vi "SECoP_dataCreateScaled.vi"(6 "value":i64, 7 "scale factor":dbl=1.0, 8 "error in (no error)":errorcluster, 9 "maximum value":i64=9223372036854775807, 10 "minimum value":i64=-9223372036854775807, 11 "DLL path (in)":T2) -> (0 "error out":errorcluster, 2 "SECoP_dataPtr (out)":T1 {"ptr64" format="%.0x"; "ptr32" format="%.0x"}, 3 "DLL path (out)":T2)   [LabVIEW 2023, in "SECoP.lvlib"]
doc: "Call <b>\"SECoP_dataCreateScaled.vi\"</b> to create a simple scaled (numeric) data type and set value. This data type is based on an integer with a scaling factor. Free resources after use with <b>\"SECoP_dataDestroy.vi\"</b>.\n\n<b>DLL path</b> input and output of cluster from \"SECoP-Initialize.vi\"\n<b>scale factor</b> scaling factor\n<b>minimum value</b> smallest allowed integer value without scaling\n<b>maximum value</b> greatest allowed integer value without scaling\n<b>value</b> new value\n<b>SECoP_dataPtr</b> created data"
uses:
  SECoP.lvlib
  SECoP-libraries.ctl
  SECoP-data.ctl
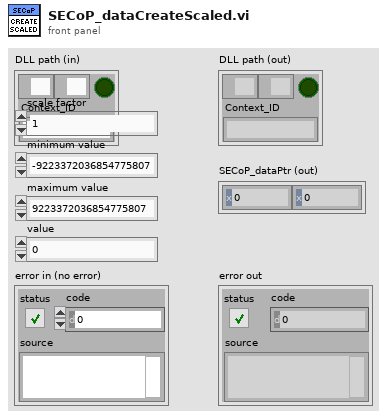
[diagram p1: front panel]
types:
  T1 = typedef "SECoP.lvlib/SECoP-data.ctl" = cluster{"ptr32":u32, "ptr64":u64}
  T2 = typedef "SECoP.lvlib/SECoP-libraries.ctl" = cluster{"serverDLL":path, "variantDLL":path, "cleanup_mode":bool, "Context_ID":string}
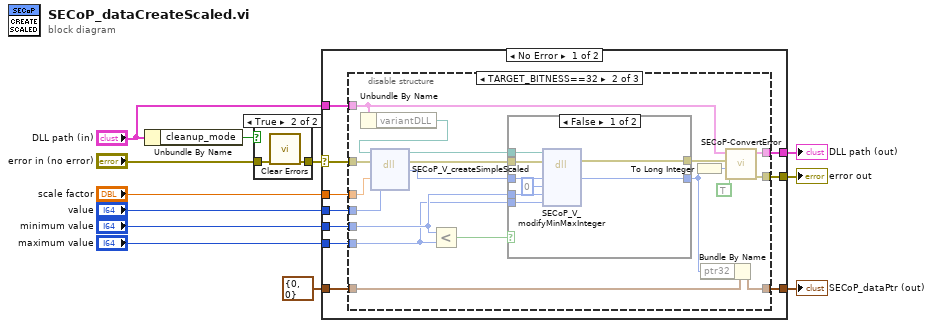
[diagram p0: block diagram]
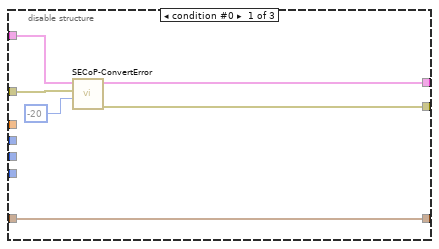
[diagram p3: hidden frame]
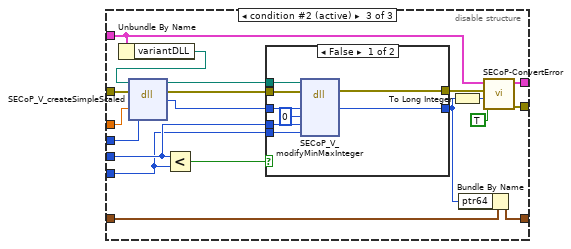
[diagram p5: hidden frame]
diagram:
  n1 = Unbundle By Name("DLL path (in)") -> ("cleanup_mode"=w10:bool)
  n2 = case shown="True" w10 {
    tunnel: "error in (no error)" -> [w13 w15]
    tunnel: [w13 w14] -> w8
    frame False {
    }
    frame True {
      n3 = call <vilib>:"Clear Errors.vi"("error in (no error)"=w15) -> ("error out"=w14:errorcluster)  [unwired: 5 in, 1 out]
    }
  }
  n4 = case shown="No Error" w8 {
    selector: w8 -> [w25 w91]
    tunnel: "DLL path (in)" -> [w24 w92]
    tunnel: [w22 w92] -> w12
    tunnel: [w23 w91] -> w11
    tunnel: [w20 w90] -> w7
    tunnel: T1 {"ptr32"=0, "ptr64"=0} ("SECoP_dataPtr (out)") -> [w21 w90]
    tunnel: "minimum value" -> [w19 _]
    tunnel: "maximum value" -> [w18 _]
    tunnel: "scale factor" -> [w17 _]
    tunnel: "value" -> [w16 _]
    frame No Error {
      n5 = disable-structure shown="TARGET_BITNESS==32" {
        disable-tunnel: w25 -> [w31 w50 w79]
        disable-tunnel: w24 -> [w30 w33 w62]
        disable-tunnel: [w28 w47 w76] -> w23
        disable-tunnel: [w29 w46 w75] -> w22
        disable-tunnel: w21 -> [w26 w48 w77]
        disable-tunnel: [w26 w49 w78] -> w20
        disable-tunnel: w19 -> [_ w38 w67]
        disable-tunnel: w18 -> [_ w37 w66]
        disable-tunnel: w17 -> [_ w35 w64]
        disable-tunnel: w16 -> [_ w34 w63]
        frame condition #0 {
          n6 = call "SECoP-ConvertError.vi"("return code"=-20, "error in (no error)"=w31, "DLL path (in)"=w30) -> ("error out"=w28:errorcluster, "DLL path (out)"=w29:T2)  [unwired: 7 in]
        }
        frame condition #1 {
          n7 = Unbundle By Name(w33) -> ("variantDLL"=w32:path)
          n8 = dll-call lib="Z:/Praktische_Aufgaben/SECoP-LabVIEW2015/32bit/SECoP32.dll" fn="SECoP_V_createSimpleScaled"(path in=w32, error in=w50, "dScale"=w35, "llValue"=w34) -> (path out=w43:path, error out=w42:errorcluster, "return type"=w40:u32)  [unwired: 3 in]
          n9 = Less?(x=w38, y=w37) -> (x < y?=w36:bool)
          n10 = case shown="False" w36 {
            tunnel: w43 -> [w58 _]
            tunnel: w42 -> [w57 w60]
            tunnel: [w56 w60] -> w41
            tunnel: w40 -> [w55 w59]
            tunnel: [w54 w59] -> w39
            tunnel: w38 -> [w52 _]
            tunnel: w37 -> [w51 _]
            frame False {
              n11 = dll-call lib="Z:/Praktische_Aufgaben/SECoP-LabVIEW2015/32bit/SECoP32.dll" fn="SECoP_V_modifyMinMaxInteger"(path in=w58, error in=w57, "pData"=w55, "uPosition"=u32 0, "llMinimum"=w52, "llMaximum"=w51) -> (error out=w56:errorcluster, "pData"=w54:u32)  [unwired: 5 in, 1 out]
            }
            frame True {
            }
          }
          n12 = To Long Integer(number=w39) -> (32bit integer=w44:i32)
          n13 = Bundle By Name(cluster=w48, "ptr32"=w39) -> (w49:T1)
          n14 = call "SECoP-ConvertError.vi"("return is boolean"=TRUE, "return code"=w44, "error in (no error)"=w41, "DLL path (in)"=w33) -> ("error out"=w47:errorcluster, "DLL path (out)"=w46:T2)  [unwired: 6 in]
        }
        frame condition #2 (active) {
          n15 = Unbundle By Name(w62) -> ("variantDLL"=w61:path)
          n16 = dll-call lib="Z:/Praktische_Aufgaben/SECoP-LabVIEW2015/32bit/SECoP32.dll" fn="SECoP_V_createSimpleScaled"(path in=w61, error in=w79, "dScale"=w64, "llValue"=w63) -> (path out=w72:path, error out=w71:errorcluster, "return type"=w69:u64)  [unwired: 3 in]
          n17 = Less?(x=w67, y=w66) -> (x < y?=w65:bool)
          n18 = case shown="False" w65 {
            tunnel: w72 -> [w87 _]
            tunnel: w71 -> [w86 w89]
            tunnel: [w85 w89] -> w70
            tunnel: w69 -> [w84 w88]
            tunnel: [w83 w88] -> w68
            tunnel: w67 -> [w81 _]
            tunnel: w66 -> [w80 _]
            frame False {
              n19 = dll-call lib="Z:/Praktische_Aufgaben/SECoP-LabVIEW2015/32bit/SECoP32.dll" fn="SECoP_V_modifyMinMaxInteger"(path in=w87, error in=w86, "pData"=w84, "uPosition"=u32 0, "llMinimum"=w81, "llMaximum"=w80) -> (error out=w85:errorcluster, "pData"=w83:u64)  [unwired: 5 in, 1 out]
            }
            frame True {
            }
          }
          n20 = To Long Integer(number=w68) -> (32bit integer=w73:i32)
          n21 = Bundle By Name(cluster=w77, "ptr64"=w68) -> (w78:T1)
          n22 = call "SECoP-ConvertError.vi"("return is boolean"=TRUE, "return code"=w73, "error in (no error)"=w70, "DLL path (in)"=w62) -> ("error out"=w76:errorcluster, "DLL path (out)"=w75:T2)  [unwired: 6 in]
        }
      }
    }
    frame Error {
    }
  }
  "DLL path (out)" <- w12
  "error out" <- w11
  "SECoP_dataPtr (out)" <- w7
